vi "Initialize.vi"(0 "VISA resource name":refnum<visa-resource-name>, 5 "ID Query (T: Check)":bool=TRUE, 7 "Reset (T: Reset)":bool=TRUE, 9 "Reset Defaults (F:Dont Reset)":bool, 11 "error in (no error)":errorcluster) -> (4 "VISA resource name out":refnum<visa-resource-name>, 15 "error out":errorcluster)   [LabVIEW 2017, in "Lake Shore Cryotronics 218.lvlib"]
doc: "This VI passes the addressing information in the instrument decriptor to the Instr Open VI and returns the instrument ID. You can optionally reset the instrument by setting the front panel reset control. You must run this VI before using any of the instrument driver VIs for this instrument.\n\nNOTE: If you do not want the instrument reset to its default setup state you MUST set the Reset Defaults control to FALSE."
uses:
  Lake Shore Cryotronics 218.lvlib
panel:
  # "© 2005 National Instruments.  ALL RIGHTS RESERVED."
  # "Check\nDon't Check"
  # "Reset\nDon't Reset"
  # "Reset to Default State\nDon't Reset to Default State"
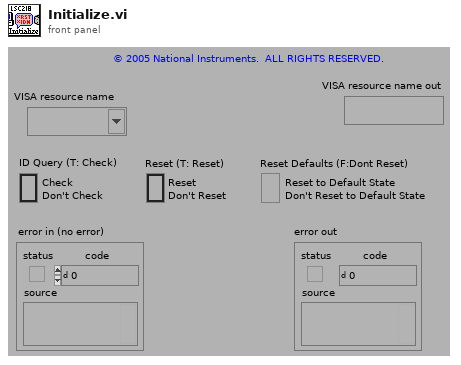
[diagram p1: front panel]
types:
  T1 = cluster{"Status":bool, "Code":i32, "Source (VI Name)":string}
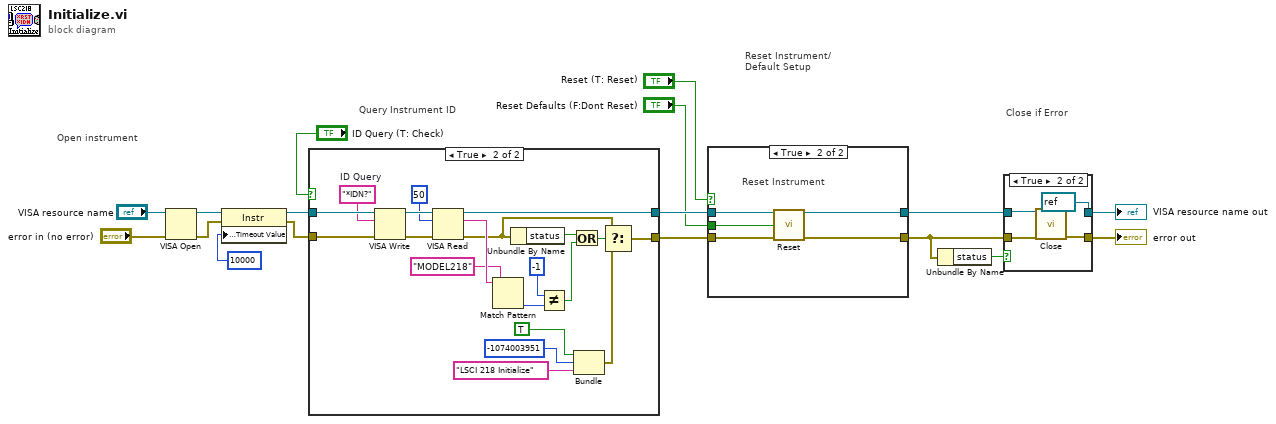
[diagram p0: block diagram]
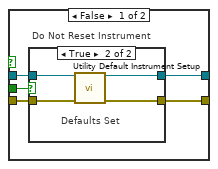
[diagram p3: hidden frame]
diagram:
  # "Close if Error"
  # "Query Instrument ID"
  # "Reset Instrument/\nDefault Setup"
  # "Open instrument"
  n1 = VISA Open(error in (no error)="error in (no error)", VISA resource name="VISA resource name") -> (VISA resource name=w4:refnum<visa-resource-name>, error out=w6:errorcluster)  [unwired: 3 in]
  n2 = property class="Instr"(reference=w4, error in=w6, "General Settings:Timeout Value"=u32 10000 ("Tmo Value")) -> (reference out=w3:refnum<visa-resource-name>, error out=w5:errorcluster)
  n3 = case shown="True" "ID Query (T: Check)" {
    tunnel: [w18 w39] -> w16
    tunnel: [w19 w36] -> w17
    tunnel: w3 -> [w19 w37]
    tunnel: w5 -> [w18 w38]
    frame False {
    }
    frame True {
      w23 = "*IDN?"  # ID Query
      n4 = VISA Write(VISA resource name=w37, write buffer=w23, error in (no error)=w38) -> (VISA resource name out=w32:refnum<visa-resource-name>, error out=w30:errorcluster)  [unwired: 1 out]
      n5 = VISA Read(VISA resource name=w32, byte count=u32 50, error in (no error)=w30) -> (VISA resource name out=w36:refnum<visa-resource-name>, read buffer=w33:string, error out=w31:errorcluster)  [unwired: 1 out]
      n6 = Match Pattern(string=w33, regular expression="MODEL218") -> (offset past match=w25:i32)  [unwired: 1 in, 3 out]
      n7 = Unbundle By Name(w31) -> ("status"=w28:bool)
      n8 = Not Equal?(x=-1, y=w25) -> (x != y?=w34:bool)
      n9 = Or(x=w28, y=w34) -> (x .or. y?=w29:bool)
      n10 = Bundle("Status"=TRUE, "Code"=-1074003951, "Source (VI Name)"="LSCI 218 Initialize") -> (w22:T1)  [unwired: 1 in]
      n11 = Select(t=w31, s=w29, f=w22) -> (s? t:f=w39:T1)
    }
  }
  n12 = case shown="True" "Reset (T: Reset)" {
    tunnel: w16 -> [w43 w52]
    tunnel: [w42 w55] -> w11
    tunnel: w17 -> [w44 w53]
    tunnel: [w41 w54] -> w10
    tunnel: "Reset Defaults (F:Dont Reset)" -> [w40 w51]
    frame False {
      # "Do Not Reset Instrument"
      n13 = case shown="True" w40 {
        tunnel: w44 -> [w46 w50]
        tunnel: w43 -> [w45 w49]
        tunnel: [w45 w48] -> w42
        tunnel: [w46 w47] -> w41
        frame False {
          # "No Defaults Set"
        }
        frame True {
          # "Defaults Set"
          n14 = call "Utility Default Instrument Setup.vi"("VISA resource name"=w50, "error in (no error)"=w49) -> ("VISA resource name out"=w47:refnum<visa-resource-name>, "error out"=w48:errorcluster)  [unwired: 12 in]
        }
      }
    }
    frame True {
      # "Reset Instrument"
      n15 = call "Reset.vi"("VISA resource name"=w53, "Reset Defaults (F:Dont Reset)"=w51, "error in (no error)"=w52) -> ("VISA resource name out"=w54:refnum<visa-resource-name>, "error out"=w55:errorcluster)  [unwired: 11 in]
    }
  }
  n16 = Unbundle By Name(w11) -> ("status"=w12:bool)
  n17 = case shown="True" w12 {
    tunnel: w10 -> [w57 w59]
    tunnel: w11 -> [w56 w61]
    tunnel: [w57 refnum<visa-resource-name> refnum ("VISA resource name out")] -> w9
    tunnel: [w56 w60] -> w8
    frame False {
    }
    frame True {
      n18 = call "Close.vi"("VISA resource name"=w59, "error in (no error)"=w61) -> ("error out"=w60:errorcluster)  [unwired: 13 in]
    }
  }
  "VISA resource name out" <- w9
  "error out" <- w8
